vi "Ballard - Arinc-429 - Main Page.vi"(8 "error in (no error)":errorcluster, 11 "Node Ptr":T2 format="%.0x") -> (0 "error out":errorcluster)   [LabVIEW 2020, in "Ballard Arinc-429 System Explorer.lvlib"]
uses:
  Ballard Arinc-429 System Explorer.lvlib
  <vilib>/NI VeriStand/Custom Device API/Custom Device Item Ref.ctl
  Shared/Controls and Global/Initialization Method.ctl
  Shared/Controls and Global/Global.vi
  <vilib>/NI VeriStand/Custom Device API/Get Item Property (U16).vi
  <vilib>/NI VeriStand/Custom Device API/Get Item Property (I32).vi
  <vilib>/NI VeriStand/Custom Device API/Get Item Property (Boolean).vi
  <vilib>/NI VeriStand/Custom Device API/Get Item Property (Path).vi
  <vilib>/NI VeriStand/Custom Device API/Get Item Property (String).vi
  <vilib>/NI VeriStand/Custom Device API/Set Item Property (I32).vi
  <vilib>/NI VeriStand/Custom Device API/Set Item Property (String).vi
  <vilib>/NI VeriStand/Custom Device API/Set Item Property (U16).vi
  <vilib>/NI VeriStand/Custom Device API/Custom Device API.lvlib
  Shared/Ballard Arinc-429 Shared.lvlib
  <vilib>/NI VeriStand/Custom Device API/Set Item Property (Boolean).vi
panel:
  in  "Help":bool
  in  "PXI Slot Number":i32=1 min=1 max=18 step=1
  in  "Initialization Method":T1
  out "Parameters Configuration Warning text":string="WARNING: The Parameters Configuration File has changed since import. If you attempt to run this system definition an error may occur. Consider refreshing the database import."
  out "Parameters Configuration File":path
  in  "Core Number":i32
  in  "Card Number":i32 min=0 max=18 step=1
  out "Version":string
  in  "ScheduledSDI?":bool
  in  "RefreshDB":bool
  out "HW Configuration Warning text":string="WARNING: The database has changed since import. If you attempt to run this system definition an error may occur. Consider refreshing the database import."
  out "Warn Icon":bool
  out "Hardware Configuration File":path
  in  "Header":cluster{"Section Name":string}={"Section Name"="Ballard - Arinc-429 -  Custom Device"}
  in  "Description":string
  in  "Name":string
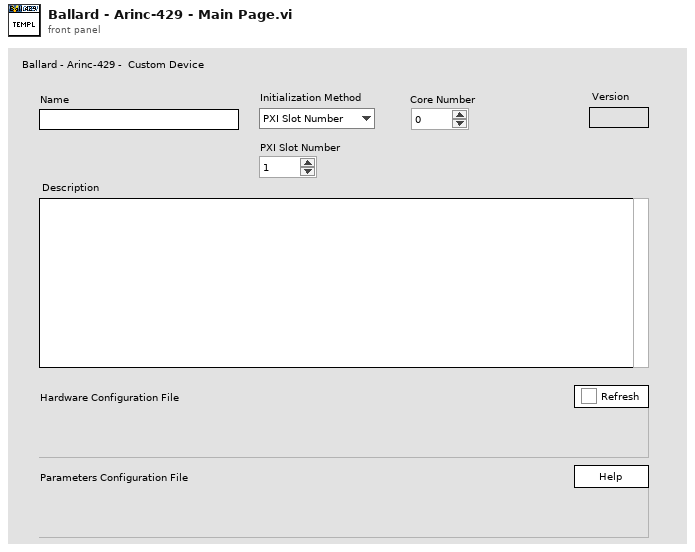
[diagram p1: front panel]
types:
  T1 = typedef "Ballard Arinc-429 Shared.lvlib/Initialization Method.ctl" = enum16{"PXI Slot Number", "Card Number"}
  T2 = typedef "Custom Device API.lvlib/Custom Device Item Ref.ctl" = u64
  T3 = typedef "Custom Device API.lvlib/Custom Device Item Info.ctl" = cluster{"Name":string, "Is Channel":bool, "GUID":string, "Is Waveform":bool}
  T4 = typedef "Custom Device API.lvlib/Custom Device Commands.ctl" = enum16{"Default", "Item renamed", "Shutdown", "Dynamic button pressed"}
  T5 = typedef "Ballard Arinc-429 System Explorer.lvlib/Refresh Match Settings.ctl" = cluster{"Ch by name?":bool, "Lbl by name?":bool}
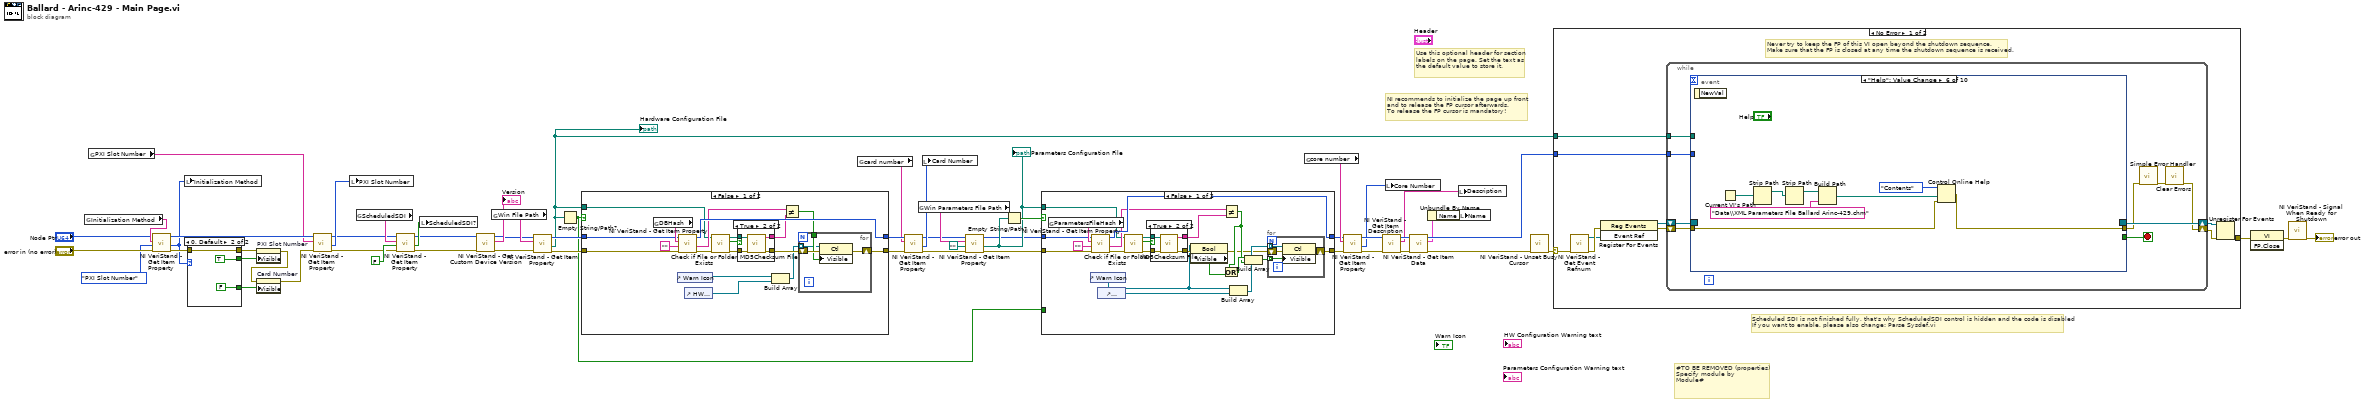
[diagram p0: block diagram]
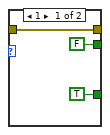
[diagram p2: hidden frame]
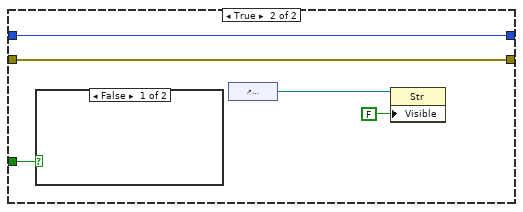
[diagram p4: hidden frame]
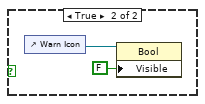
[diagram p5: hidden frame]
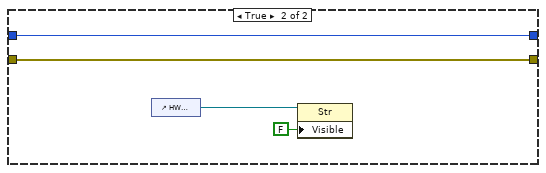
[diagram p7: hidden frame]
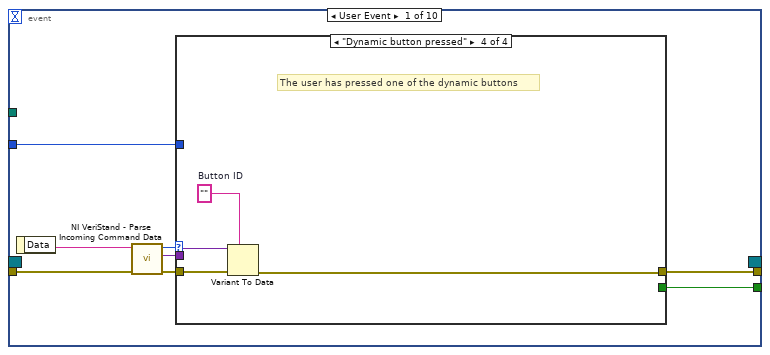
[diagram p8: hidden frame]
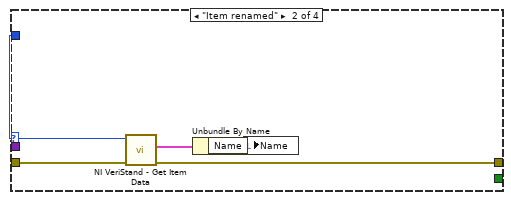
[diagram p10: hidden frame]
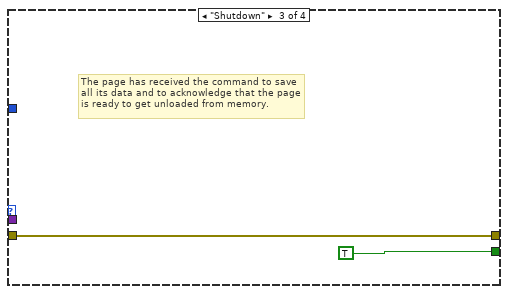
[diagram p11: hidden frame]
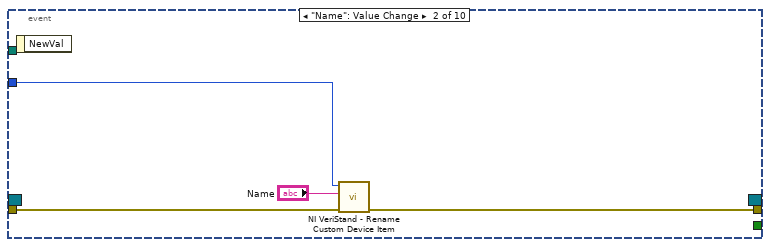
[diagram p12: hidden frame]
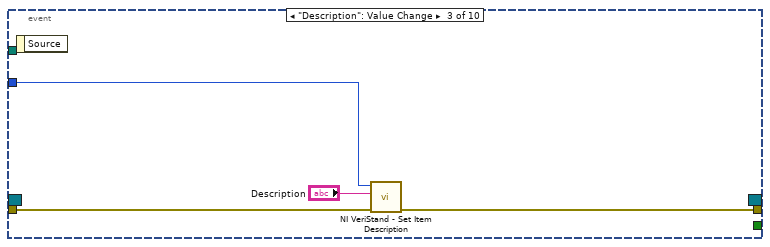
[diagram p13: hidden frame]
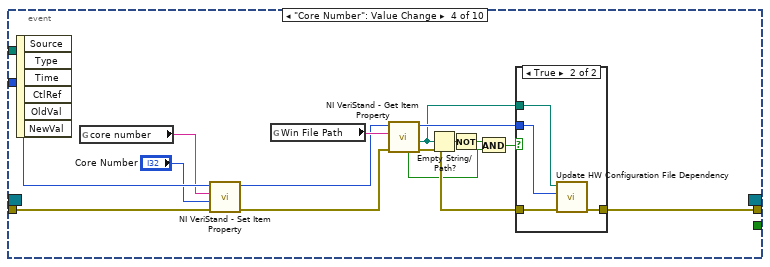
[diagram p14: hidden frame]
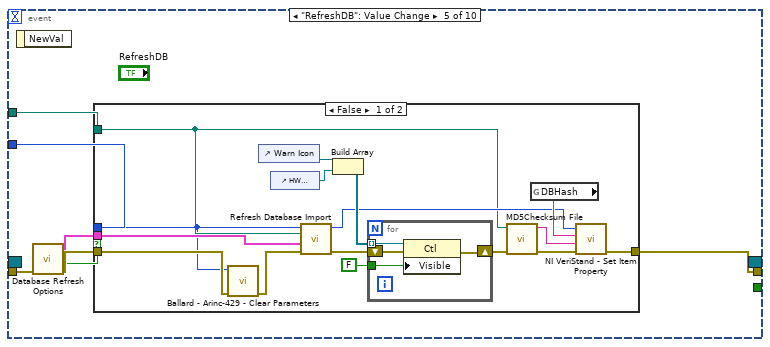
[diagram p16: hidden frame]
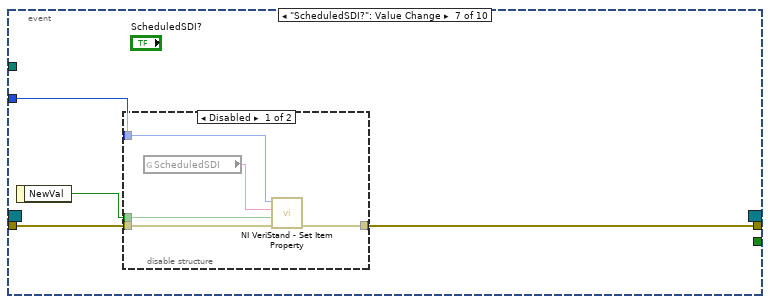
[diagram p18: hidden frame]
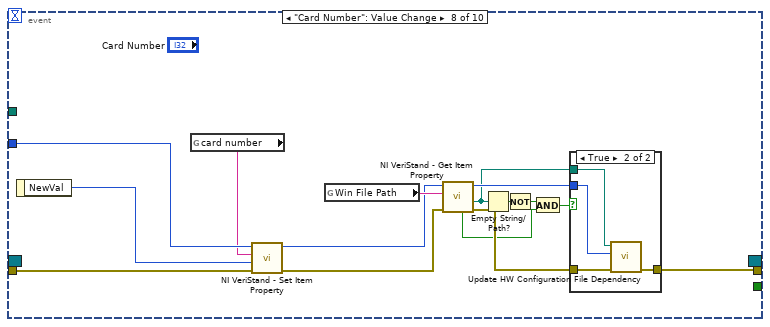
[diagram p20: hidden frame]
diagram:
  # "#TO BE REMOVED (properties)\nSpecify module by\nModule#"
  # "Scheduled SDI is not finished fully, that's why ScheduledSDI control is hidden and the code is disabled\nIf you want to enable, please also change: Parse Sysdef.vi"
  # "Use this optional header for section labels on the page. Set the text as the default value to store it."
  # "NI recommends to initialize the page up front\nand to release the FP cursor afterwards.\nTo release the FP cursor is mandatory!"
  n1 = global read "Global.vi" "Initialization Method"() -> (w16:string)
  n2 = global read "Global.vi" "PXI Slot Number"() -> (w14:string)
  n3 = call-poly <vilib>:"NI VeriStand - Get Item Property.vi"("error in (no error)"="error in (no error)", "Default Value"=Initialization_Method."PXI Slot Number" ("Initialization Method"), "Property Name"=w16, "Item Ref in"="Node Ptr") -> ("error out"=w7:errorcluster, "Value"=w6:u16, "Item Ref out"=w15:T2)  [unwired: 4 in, 1 out]
  n4 = local write "Initialization Method"(w6) -> ()
  n5 = case shown="0, Default" w6 {
    tunnel: w7 -> [w61 w64]
    tunnel: [FALSE TRUE] -> w5
    tunnel: [w61 w64] -> w4
    tunnel: [TRUE FALSE] -> w1
    frame 1 {
    }
    frame 0, Default {
    }
  }
  n6 = property on="PXI Slot Number" class="DigNum (strict)"(error in=w4, "Visible"=w5) -> (error out=w3:errorcluster)  [unwired: 1 in, 1 out]
  n7 = property on="Card Number" class="DigNum (strict)"(error in=w3, "Visible"=w1) -> (error out=w2:errorcluster)  [unwired: 1 in, 1 out]
  n8 = call-poly <vilib>:"NI VeriStand - Get Item Property.vi"("error in (no error)"=w2, "Property Name"=w14, "Item Ref in"=w15) -> ("error out"=w8:errorcluster, "Value"=w10:i32, "Item Ref out"=w9:T2)  [unwired: 5 in, 1 out]
  n9 = local write "PXI Slot Number"(w10) -> ()
  n10 = global read "Global.vi" "ScheduledSDI"() -> (w40:string)
  n11 = call-poly <vilib>:"NI VeriStand - Get Item Property.vi"("error in (no error)"=w8, "Default Value"=FALSE, "Property Name"=w40, "Item Ref in"=w9) -> ("error out"=w41:errorcluster, "Value"=w38:bool, "Item Ref out"=w37:T2)  [unwired: 4 in, 1 out]
  n12 = local write "ScheduledSDI?"(w38) -> ()
  n13 = call <vilib>:"NI VeriStand - Get Custom Device Version.vi"("error in (no error)"=w41, "Device Ref in"=w37) -> ("error out"=w34:errorcluster, "Value"=→"Version":string, "Device Ref out"=w35:T2)  [unwired: 7 in]
  n14 = global read "Global.vi" "Win File Path"() -> (w47:string)
  n15 = call-poly <vilib>:"NI VeriStand - Get Item Property.vi"("error in (no error)"=w34, "Property Name"=w47, "Item Ref in"=w35) -> ("error out"=w46:errorcluster, "Value"=w42:path, "Item Ref out"=w43:T2)  [unwired: 5 in, 1 out]
  "Hardware Configuration File" <- w42
  n16 = Empty String/Path?(string/path=w42) -> (empty?=w17:bool)
  n17 = case shown="False" w17 {
    tunnel: w46 -> [w79 w95]
    tunnel: [w70 w95] -> w45
    tunnel: [w78 w94] -> w44
    tunnel: w43 -> [w80 w94]
    tunnel: w42 -> [w66 _]
    frame False {
      n18 = global read "Global.vi" "DBHash"() -> (w81:string)
      n19 = control-ref of="Warn Icon"() -> (w72:refnum<vi>)
      n20 = call-poly <vilib>:"NI VeriStand - Get Item Property.vi"("error in (no error)"=w79, "Default Value"="", "Property Name"=w81, "Item Ref in"=w80) -> ("error out"=w67:errorcluster, "Value"=w76:string, "Item Ref out"=w78:T2)  [unwired: 4 in, 1 out]
      n21 = control-ref of="HW Configuration Warning text"() -> (w73:refnum<vi>)
      n22 = call <vilib>:"Check if File or Folder Exists.vi"("error in (no error)"=w67, "path"=w66) -> ("error out"=w69:errorcluster, "file or folder exists?"=w65:bool, "dup path"=w68:path)  [unwired: 7 in]
      n23 = case shown="True" w65 {
        tunnel: [_ w87] -> w77
        tunnel: [w83 w86] -> w75
        tunnel: w69 -> [w83 w85]
        tunnel: w68 -> [_ w84]
        frame False {
        }
        frame True {
          n24 = call <vilib>:"MD5Checksum File.vi"("error in (no error)"=w85, "Path"=w84) -> ("error out"=w86:errorcluster, "MD5 message-digest"=w87:string)  [unwired: 8 in]
        }
      }
      n25 = Build Array(w72, w73) -> (w71:refnum<vi>[])
      n26 = Not Equal?(x=w76, y=w77) -> (x != y?=w74:bool)
      n27 = for {
        shift-right: [w90] -> w70
        shift-left: w75 -> [w91]
        tunnel: w74 -> [w89]
        tunnel: w71 -> [w88] mode=indexing
        n28 = property class="Ctl"(reference=w88, error in=w91, "Visible"=w89) -> (error out=w90:errorcluster)  [unwired: 1 out]
      }
    }
    frame True {
      n29 = control-ref of="HW Configuration Warning text"() -> (w93:refnum<vi>)
      n30 = property class="Str"(reference=w93, "Visible"=FALSE) -> ()  [unwired: 1 in, 2 out]
    }
  }
  n31 = global read "Global.vi" "card number"() -> (w29:string)
  n32 = call-poly <vilib>:"NI VeriStand - Get Item Property.vi"("error in (no error)"=w45, "Property Name"=w29, "Item Ref in"=w44) -> ("error out"=w25:errorcluster, "Value"=w28:i32, "Item Ref out"=w26:T2)  [unwired: 5 in, 1 out]
  n33 = global read "Global.vi" "Win Parameters File Path"() -> (w27:string)
  n34 = local write "Card Number"(w28) -> ()
  n35 = call-poly <vilib>:"NI VeriStand - Get Item Property.vi"("error in (no error)"=w25, "Default Value"=path "", "Property Name"=w27, "Item Ref in"=w26) -> ("error out"=w20:errorcluster, "Value"=w23:path, "Item Ref out"=w22:T2)  [unwired: 4 in, 1 out]
  "Parameters Configuration File" <- w23
  n36 = Empty String/Path?(string/path=w23) -> (empty?=w24:bool)
  n37 = case shown="False" w24 {
    tunnel: [w111 w130] -> w19
    tunnel: [w114 w131] -> w21
    tunnel: w22 -> [w115 w131]
    tunnel: w23 -> [w107 _]
    tunnel: w20 -> [w96 w130]
    tunnel: w17 -> [_ w127]
    frame False {
      n38 = global read "Global.vi" "ParametersFileHash"() -> (w116:string)
      n39 = control-ref of="Warn Icon"() -> (w97:refnum<vi>)
      n40 = call-poly <vilib>:"NI VeriStand - Get Item Property.vi"("error in (no error)"=w96, "Default Value"="", "Property Name"=w116, "Item Ref in"=w115) -> ("error out"=w108:errorcluster, "Value"=w112:string, "Item Ref out"=w114:T2)  [unwired: 4 in, 1 out]
      n41 = control-ref of="Parameters Configuration Warning text"() -> (w105:refnum<vi>)
      n42 = call <vilib>:"Check if File or Folder Exists.vi"("error in (no error)"=w108, "path"=w107) -> ("error out"=w110:errorcluster, "file or folder exists?"=w106:bool, "dup path"=w109:path)  [unwired: 7 in]
      n43 = case shown="True" w106 {
        tunnel: [_ w126] -> w113
        tunnel: [w122 w125] -> w102
        tunnel: w110 -> [w122 w124]
        tunnel: w109 -> [_ w123]
        frame False {
        }
        frame True {
          n44 = call <vilib>:"MD5Checksum File.vi"("error in (no error)"=w124, "Path"=w123) -> ("error out"=w125:errorcluster, "MD5 message-digest"=w126:string)  [unwired: 8 in]
        }
      }
      n45 = property class="Bool"(reference=w97, error in=w102) -> (error out=w98:errorcluster, "Visible"=w100:bool)  [unwired: 1 out]
      n46 = Not Equal?(x=w112, y=w113) -> (x != y?=w99:bool)
      n47 = Or(x=w99, y=w100) -> (x .or. y?=w101:bool)
      n48 = Build Array(w97, w105) -> (w104:refnum<vi>[])
      n49 = Build Array(w101, w99) -> (w103:bool[])
      n50 = for {
        tunnel: w103 -> [w119] mode=indexing
        shift-right: [w120] -> w111
        shift-left: w98 -> [w121]
        tunnel: w104 -> [w118] mode=indexing
        n51 = property class="Ctl"(reference=w118, error in=w121, "Visible"=w119) -> (error out=w120:errorcluster)  [unwired: 1 out]
      }
    }
    frame True {
      n52 = case shown="False" w127 {
        frame False {
        }
        frame True {
          n53 = control-ref of="Warn Icon"() -> (w133:refnum<vi>)
          n54 = property class="Bool"(reference=w133, "Visible"=FALSE) -> ()  [unwired: 1 in, 2 out]
        }
      }
      n55 = control-ref of="Parameters Configuration Warning text"() -> (w129:refnum<vi>)
      n56 = property class="Str"(reference=w129, "Visible"=FALSE) -> ()  [unwired: 1 in, 2 out]
    }
  }
  n57 = global read "Global.vi" "core number"() -> (w30:string)
  n58 = call-poly <vilib>:"NI VeriStand - Get Item Property.vi"("error in (no error)"=w19, "Property Name"=w30, "Item Ref in"=w21) -> ("error out"=w33:errorcluster, "Value"=w31:i32, "Item Ref out"=w32:T2)  [unwired: 5 in, 1 out]
  n59 = call <vilib>:"NI VeriStand - Get Item Description.vi"("error in (no error)"=w33, "Item Ref in"=w32) -> ("error out"=w50:errorcluster, "Description"=w51:string, "Item Ref out"=w52:T2)  [unwired: 7 out]
  n60 = local write "Core Number"(w31) -> ()
  n61 = call <vilib>:"NI VeriStand - Get Item Data.vi"("error in (no error)"=w50, "Item Ref in"=w52) -> ("error out"=w55:errorcluster, "Item Info"=w49:T3, "Item Ref out"=w53:T2)  [unwired: 7 out]
  n62 = Unbundle By Name(w49) -> ("Name"=w48:string)
  n63 = local write "Description"(w51) -> ()
  n64 = local write "Name"(w48) -> ()
  n65 = call <vilib>:"NI VeriStand - Unset Busy Cursor.vi"("error in (no error)"=w55) -> ("error out"=w54:errorcluster)  [unwired: 10 out]
  n66 = case shown="No Error" w54 {
    selector: w54 -> [w135 w305]
    tunnel: [w140 w303] -> w58
    tunnel: w53 -> [w136 _]
    tunnel: w42 -> [w134 _]
    frame No Error {
      # "Never try to keep the FP of this VI open beyond the shutdown sequence.\nMake sure that the FP is closed at any time the shutdown sequence is received."
      n67 = call <vilib>:"NI VeriStand - Get Event Refnum.vi"("error in (no error)"=w135) -> ("error out"=w143:errorcluster, "Event Ref"=w139:refnum<user-event>)  [unwired: 9 out]
      n68 = register-events(error in=w143, w139) -> (reference out=w137:refnum<event-registration>, error out=w138:errorcluster)  [unwired: 1 in]
      n69 = while {
        tunnel: w136 -> [w148]
        shift-right: [w145] -> w141
        shift-left: w138 -> [w151]
        shift-right: [w152] -> w142
        shift-left: w137 -> [w150]
        tunnel: w134 -> [w144]
        stop <- w149 stop-if-true
        n70 = event shown="[5] \"Help\": Value Change" {
          selector: w150 -> [_ _ _ _ _ _ _ _ _ _]
          dyn-events: [_ _ _ _ _ _ _ _ _ _] -> w152
          timeout: _ -> [_ _ _ _ _ _ _ _ _ _]
          tunnel: w151 -> [w160 w176 w179 w195 w202 w235 w240 w261 w281 w296]
          tunnel: [w156 _ _ _ _ _ _ _ _ _] -> w149
          tunnel: [w155 w175 w178 w182 w201 w234 w237 w252 w272 w287] -> w147
          tunnel: w148 -> [w154 w174 w180 w194 w206 _ w239 w260 w280 w291]
          tunnel: w144 -> [_ _ _ _ w207 _ _ _ _ _]
          event User Event {
            n71 = event-data() -> ("Data"=w159:string)  [unwired: 1 out]
            n72 = call <vilib>:"NI VeriStand - Parse Incoming Command Data.vi"("error in (no error)"=w160, "Incoming data"=w159) -> ("error out"=w158:errorcluster, "Outgoing data"=w153:variant, "Action"=w157:T4)  [unwired: 7 out]
            n73 = case shown="\"Dynamic button pressed\"" w157 {
              tunnel: w158 -> [w161 w166 w167 w172]
              tunnel: [_ _ TRUE _] -> w156
              tunnel: [w161 w163 w167 w169] -> w155
              tunnel: w154 -> [_ w165 _ _]
              tunnel: w153 -> [_ _ _ w171]
              frame "Default", Default {
              }
              frame "Item renamed" {
                n74 = call <vilib>:"NI VeriStand - Get Item Data.vi"("error in (no error)"=w166, "Item Ref in"=w165) -> ("error out"=w163:errorcluster, "Item Info"=w164:T3)  [unwired: 8 out]
                n75 = Unbundle By Name(w164) -> ("Name"=w162:string)
                n76 = local write "Name"(w162) -> ()
              }
              frame "Shutdown" {
                # "The page has received the command to save all its data and to acknowledge that the page is ready to get unloaded from memory."
              }
              frame "Dynamic button pressed" {
                w170 = ""  # Button ID
                # "The user has pressed one of the dynamic buttons"
                n77 = Variant To Data(error in=w172, type=w170, Variant=w171) -> (error out=w169:errorcluster)  [unwired: 1 out]
              }
            }
          }
          event "Name": Value Change {
            n78 = event-data() -> ()  [unwired: 2 out]
            n79 = call <vilib>:"NI VeriStand - Rename Custom Device Item.vi"("error in (no error)"=w176, "New Name"="Name", "Item Ref in"=w174) -> ("error out"=w175:errorcluster)  [unwired: 1 in, 7 out]
          }
          event "Description": Value Change {
            n80 = event-data() -> ()  [unwired: 2 out]
            n81 = call <vilib>:"NI VeriStand - Set Item Description.vi"("error in (no error)"=w179, "Description"="Description", "Item Ref in"=w180) -> ("error out"=w178:errorcluster)  [unwired: 8 out]
          }
          event "Core Number": Value Change {
            n82 = event-data() -> ()  [unwired: 7 out]
            n83 = global read "Global.vi" "core number"() -> (w192:string)
            n84 = call-poly <vilib>:"NI VeriStand - Set Item Property.vi"("error in (no error)"=w195, "Value"="Core Number", "Property Name"=w192, "Item Ref in"=w194) -> ("error out"=w184:errorcluster, "Item Ref out"=w183:T2)  [unwired: 5 in, 1 out]
            n85 = global read "Global.vi" "Win File Path"() -> (w191:string)
            n86 = call-poly <vilib>:"NI VeriStand - Get Item Property.vi"("error in (no error)"=w184, "Property Name"=w191, "Item Ref in"=w183) -> ("error out"=w190:errorcluster, "Value"=w181:path, "Item Ref out"=w189:T2, "Found?"=w187:bool)  [unwired: 5 in]
            n87 = Empty String/Path?(string/path=w181) -> (empty?=w188:bool)
            n88 = Not(x=w188) -> (.not. x?=w185:bool)
            n89 = And(x=w185, y=w187) -> (x .and. y?=w186:bool)
            n90 = case shown="True" w186 {
              tunnel: [w196 w200] -> w182
              tunnel: w190 -> [w196 w199]
              tunnel: w189 -> [_ w198]
              tunnel: w181 -> [_ w197]
              frame False {
              }
              frame True {
                n91 = call "Update HW Configuration File Dependency.vi"("error in (no error)"=w199, "Node Ptr dup"=w198, "selected path in"=w197) -> ("error out"=w200:errorcluster)  [unwired: 8 in]
              }
            }
          }
          event "RefreshDB": Value Change {
            n92 = event-data() -> ()  [unwired: 2 out]
            n93 = call "Database Refresh Options.vi"("error in (no error)"=w202) -> ("error out"=w205:errorcluster, "Cancelled?"=w204:bool, "Refresh Settings"=w203:T5)  [unwired: 8 in]
            n94 = case shown="False" w204 {
              tunnel: [w211 w228] -> w201
              tunnel: w205 -> [w210 w228]
              tunnel: w207 -> [w213 _]
              tunnel: w206 -> [w209 _]
              tunnel: w203 -> [w212 _]
              frame False {
                n95 = call "Ballard - Arinc-429 - Clear Parameters.vi"("error in (no error)"=w210, "Node Ptr"=w209) -> ("error out"=w208:errorcluster)  [unwired: 9 in]
                n96 = control-ref of="Warn Icon"() -> (w219:refnum<vi>)
                n97 = control-ref of="HW Configuration Warning text"() -> (w220:refnum<vi>)
                n98 = call "Refresh Database Import.vi"("error in (no error)"=w208, "Match settings"=w212, "DB"=w213, "Item Ref in"=w209) -> ("error out"=w215:errorcluster, "Item Ref dup"=w214:T2)  [unwired: 5 in, 1 out]
                n99 = Build Array(w219, w220) -> (w217:refnum<vi>[])
                n100 = for {
                  shift-right: [w226] -> w218
                  shift-left: w215 -> [w227]
                  tunnel: w217 -> [w225] mode=indexing
                  tunnel: FALSE ("Visible") -> [w224]
                  n101 = property class="Ctl"(reference=w225, error in=w227, "Visible"=w224) -> (error out=w226:errorcluster)  [unwired: 1 out]
                }
                n102 = call <vilib>:"MD5Checksum File.vi"("error in (no error)"=w218, "Path"=w213) -> ("error out"=w223:errorcluster, "MD5 message-digest"=w222:string)  [unwired: 8 in]
                n103 = global read "Global.vi" "DBHash"() -> (w221:string)
                n104 = call-poly <vilib>:"NI VeriStand - Set Item Property.vi"("error in (no error)"=w223, "Value"=w222, "Property Name"=w221, "Item Ref in"=w214) -> ("error out"=w211:errorcluster)  [unwired: 5 in, 2 out]
              }
              frame True {
              }
            }
          }
          event "Help": Value Change {
            n105 = event-data() -> ()  [unwired: 2 out]
            n106 = Current VI's Path() -> (path=w233:path)
            n107 = Strip Path(path=w233) -> (stripped path=w232:path)  [unwired: 1 out]
            n108 = Strip Path(path=w232) -> (stripped path=w231:path)  [unwired: 1 out]
            n109 = Build Path(base path=w231, name or relative path="Data\\XML Parameters File Ballard Arinc-429.chm") -> (appended path=w229:path)
            n110 = Control Online Help(1:w235, 2:w229, 4:enum16{"Contents", "Key", "Close"}."Contents" ("Operation")) -> (0:w234:errorcluster)  [unwired: 1 in]
          }
          event "ScheduledSDI?": Value Change {
            n111 = event-data() -> ("NewVal"=w238:bool)  [unwired: 1 out]
            n112 = disable-structure shown="Disabled" {
              disable-tunnel: w240 -> [w245 w246]
              disable-tunnel: w239 -> [w244 _]
              disable-tunnel: w238 -> [w243 _]
              disable-tunnel: [w242 w246] -> w237
              frame Disabled {
                n113 = global read "Global.vi" "ScheduledSDI"() -> (w241:string)
                n114 = call-poly <vilib>:"NI VeriStand - Set Item Property.vi"("error in (no error)"=w245, "Value"=w243, "Property Name"=w241, "Item Ref in"=w244) -> ("error out"=w242:errorcluster)  [unwired: 5 in, 2 out]
              }
              frame Enabled {
              }
            }
          }
          event "Card Number": Value Change {
            n115 = event-data() -> ("NewVal"=w259:i32)  [unwired: 1 out]
            n116 = global read "Global.vi" "card number"() -> (w258:string)
            n117 = call-poly <vilib>:"NI VeriStand - Set Item Property.vi"("error in (no error)"=w261, "Value"=w259, "Property Name"=w258, "Item Ref in"=w260) -> ("error out"=w254:errorcluster, "Item Ref out"=w253:T2)  [unwired: 5 in, 1 out]
            n118 = global read "Global.vi" "Win File Path"() -> (w257:string)
            n119 = call-poly <vilib>:"NI VeriStand - Get Item Property.vi"("error in (no error)"=w254, "Property Name"=w257, "Item Ref in"=w253) -> ("error out"=w256:errorcluster, "Value"=w247:path, "Item Ref out"=w255:T2, "Found?"=w250:bool)  [unwired: 5 in]
            n120 = Empty String/Path?(string/path=w247) -> (empty?=w251:bool)
            n121 = Not(x=w251) -> (.not. x?=w248:bool)
            n122 = And(x=w248, y=w250) -> (x .and. y?=w249:bool)
            n123 = case shown="True" w249 {
              tunnel: [w262 w266] -> w252
              tunnel: w256 -> [w262 w265]
              tunnel: w255 -> [_ w264]
              tunnel: w247 -> [_ w263]
              frame False {
              }
              frame True {
                n124 = call "Update HW Configuration File Dependency.vi"("error in (no error)"=w265, "Node Ptr dup"=w264, "selected path in"=w263) -> ("error out"=w266:errorcluster)  [unwired: 8 in]
              }
            }
          }
          event "PXI Slot Number": Value Change {
            n125 = event-data() -> ("NewVal"=w279:i32)  [unwired: 1 out]
            n126 = global read "Global.vi" "PXI Slot Number"() -> (w278:string)
            n127 = call-poly <vilib>:"NI VeriStand - Set Item Property.vi"("error in (no error)"=w281, "Value"=w279, "Property Name"=w278, "Item Ref in"=w280) -> ("error out"=w274:errorcluster, "Item Ref out"=w273:T2)  [unwired: 5 in, 1 out]
            n128 = global read "Global.vi" "Win File Path"() -> (w277:string)
            n129 = call-poly <vilib>:"NI VeriStand - Get Item Property.vi"("error in (no error)"=w274, "Property Name"=w277, "Item Ref in"=w273) -> ("error out"=w276:errorcluster, "Value"=w267:path, "Item Ref out"=w275:T2, "Found?"=w270:bool)  [unwired: 5 in]
            n130 = Empty String/Path?(string/path=w267) -> (empty?=w271:bool)
            n131 = Not(x=w271) -> (.not. x?=w268:bool)
            n132 = And(x=w268, y=w270) -> (x .and. y?=w269:bool)
            n133 = case shown="True" w269 {
              tunnel: [w282 w286] -> w272
              tunnel: w276 -> [w282 w285]
              tunnel: w275 -> [_ w284]
              tunnel: w267 -> [_ w283]
              frame False {
              }
              frame True {
                n134 = call "Update HW Configuration File Dependency.vi"("error in (no error)"=w285, "Node Ptr dup"=w284, "selected path in"=w283) -> ("error out"=w286:errorcluster)  [unwired: 8 in]
              }
            }
          }
          event Value Change {
            n135 = event-data() -> ("NewVal"=w290:T1)  [unwired: 1 out]
            n136 = case shown="\"Card Number\"" w290 {
              tunnel: w296 -> [w299 w302]
              tunnel: [w299 w302] -> w295
              tunnel: [FALSE TRUE] -> w293
              tunnel: [TRUE FALSE] -> w292
              frame "PXI Slot Number", Default {
              }
              frame "Card Number" {
              }
            }
            n137 = property on="PXI Slot Number" class="DigNum (strict)"(error in=w295, "Visible"=w292) -> (error out=w294:errorcluster)  [unwired: 1 in, 1 out]
            n138 = property on="Card Number" class="DigNum (strict)"(error in=w294, "Visible"=w293) -> (error out=w288:errorcluster)  [unwired: 1 in, 1 out]
            n139 = global read "Global.vi" "Initialization Method"() -> (w289:string)
            n140 = call-poly <vilib>:"NI VeriStand - Set Item Property.vi"("error in (no error)"=w288, "Value"=w290, "Property Name"=w289, "Item Ref in"=w291) -> ("error out"=w287:errorcluster)  [unwired: 5 in, 2 out]
          }
        }
        n141 = call <vilib>:"Simple Error Handler.vi"("error in (no error)"=w147) -> ("error out"=w146:errorcluster)  [unwired: 1 in, 7 out]
        n142 = call <vilib>:"Clear Errors.vi"("error in (no error)"=w146) -> ("error out"=w145:errorcluster)  [unwired: 1 in, 5 out]
      }
      n143 = Unregister For Events(event registration refnum=w142, error in=w141) -> (error out=w140:errorcluster)
    }
    frame Error {
      n144 = call <vilib>:"Simple Error Handler.vi"("error in (no error)"=w305) -> ("error out"=w304:errorcluster)  [unwired: 1 in, 7 out]
      n145 = call <vilib>:"Clear Errors.vi"("error in (no error)"=w304) -> ("error out"=w303:errorcluster)  [unwired: 1 in, 5 out]
    }
  }
  n146 = invoke class="VI" method="FP.Close"(error in=w58) -> (error out=w57:errorcluster)  [unwired: 2 in, 2 out]
  n147 = call <vilib>:"NI VeriStand - Signal When Ready for Shutdown.vi"("error in (no error)"=w57) -> ("error out"=→"error out":errorcluster)  [unwired: 10 out]
